vi "Init.vi"(8 "error in":errorcluster, 10 "Sourcegrid Container":refnum<k24>(container), 11 "PDO Grid in":refnum<class "PDO Grid.lvclass">) -> (0 "error out":errorcluster, 3 "PDO Grid out":refnum<class "PDO Grid.lvclass">)   [LabVIEW 2019, in "PDO Grid.lvlib" / "PDO Grid.lvclass"]
uses:
  PDO Grid.lvclass
  D:/git/Sourcegrid-LabVIEW/source/Grid/SourceGrid.lvclass
  D:/git/Sourcegrid-LabVIEW/dll/SourceGrid.dll
  Sourcegrid-LabVIEW/dll/SourceGrid.dll
  PDO Mapping ColumnHeader/PDO Mapping Column Header.lvclass
  D:/git/Sourcegrid-LabVIEW/source/Cells/Cell/Cell.lvclass
  Sourcegrid-LabVIEW/source/Grid/SourceGrid.lvclass
  Sourcegrid-LabVIEW/source/System.Drawing.Color.ctl
  Sourcegrid-LabVIEW/source/SourceGrid.lvlib
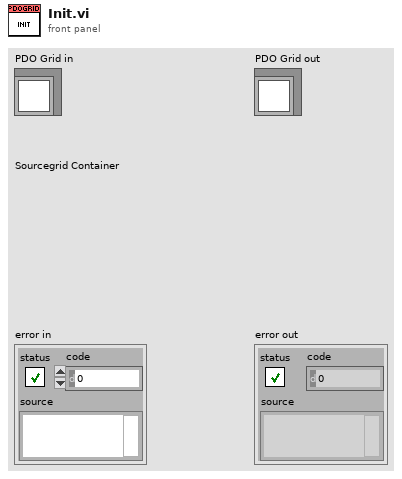
[diagram p1: front panel]
types:
  T1 = typedef "SourceGrid.lvlib/System.Drawing.Color.ctl" = enum16{"AliceBlue", "AntiqueWhite", "Aqua", "Aquamarine", "Azure", "Beige", "Bisque", "Black", "BlanchedAlmond", "Blue", "BlueViolet", "Brown", "BurlyWood", "CadetBlue", "Chartreuse", "Chocolate", "Coral", "CornflowerBlue", "Cornsilk", "Crimson", "Cyan", "DarkBlue", "DarkCyan", "DarkGoldenrod", "DarkGray", "DarkGreen", "DarkKhaki", "DarkMagenta", "DarkOliveGreen", "DarkOrange", "DarkOrchid", "DarkRed", "DarkSalmon", "DarkSeaGreen", "DarkSlateBlue", "DarkSlateGray", "DarkTurquoise", "DarkViolet", "DeepPink", "DeepSkyBlue", "DimGray", "DodgerBlue", "Firebrick", "FloralWhite", "ForestGreen", "Fuchsia", "Gainsboro", "GhostWhite", "Gold", "Goldenrod", "Gray", "Green", "GreenYellow", "Honeydew", "HotPink", "IndianRed", "Indigo", "Ivory", "Khaki", "Lavender", "LavenderBlush", "LawnGreen", "LemonChiffon", "LightBlue", "LightCoral", "LightCyan", "LightGoldenrodYellow", "LightGray", "LightGreen", "LightPink", "LightSalmon", "LightSeaGreen", "LightSkyBlue", "LightSlateGray", "LightSteelBlue", "LightYellow", "Lime", "LimeGreen", "Linen", "Magenta", "Maroon", "MediumAquamarine", "MediumBlue", "MediumOrchid", "MediumPurple", "MediumSeaGreen", "MediumSlateBlue", "MediumSpringGreen", "MediumTurquoise", "MediumVioletRed", "MidnightBlue", "MintCream", "MistyRose", "Moccasin", "NavajoWhite", "Navy", "OldLace", "Olive", "OliveDrab", "Orange", "OrangeRed", "Orchid", "PaleGoldenrod", "PaleGreen", "PaleTurquoise", "PaleVioletRed", "PapayaWhip", "PeachPuff", "Peru", "Pink", "Plum", "PowderBlue", "Purple", "Red", "RosyBrown", "RoyalBlue", "SaddleBrown", "Salmon", "SandyBrown", "SeaGreen", "SeaShell", "Sienna", "Silver", "SkyBlue", "SlateBlue", "SlateGray", "Snow", "SpringGreen", "SteelBlue", "Tan", "Teal", "Thistle", "Tomato", "Transparent", "Turquoise", "Violet", "Wheat", "White", "WhiteSmoke", "Yellow"}
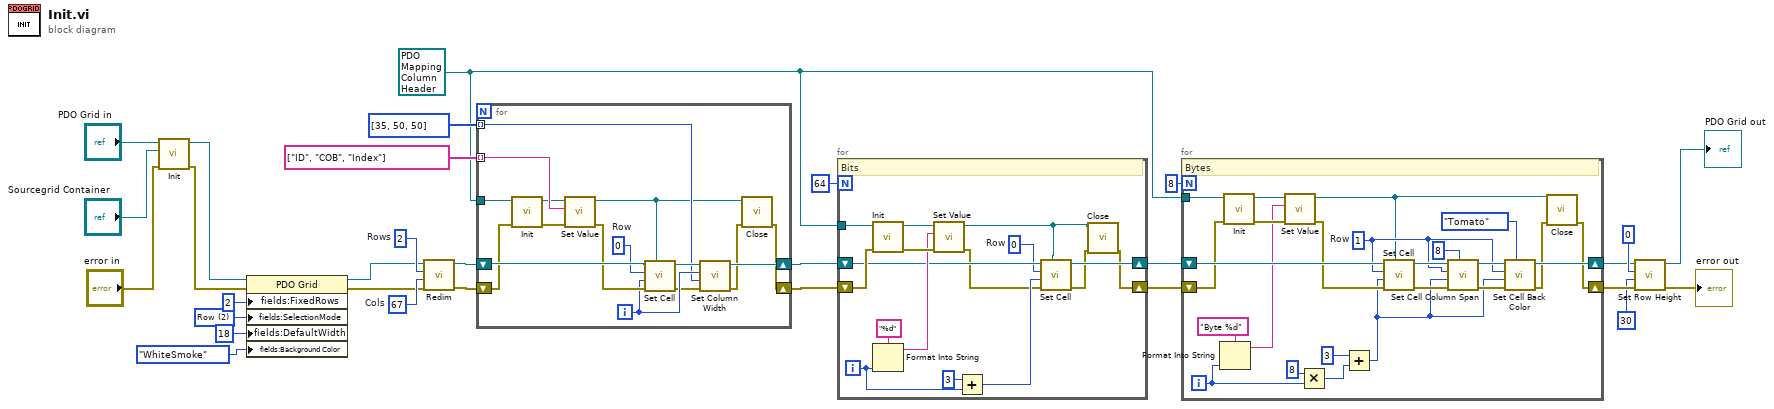
[diagram p0: block diagram]
diagram:
  w1 = refnum<class "PDO Mapping Column Header.lvclass"> refnum ("UI Actor.lvlib:PDOMapping ColumnHeader.lvclass")
  w28 = 2 items=["Cell"=1, "Row"=2, "Column"=3] ("SelectionMode")
  w29 = 67  # Cols
  w30 = 2  # Rows
  n1 = call-parent "Init.vi"("error in"="error in", "Sourcegrid Container"="Sourcegrid Container", "Grid in"="PDO Grid in") -> ("error out"=w4:errorcluster, "Grid out"=w7:refnum<class "PDO Grid.lvclass">)  [unwired: 7 in]
  n2 = property class="PDO Grid"(reference=w7, error in=w4, "fields:FixedRows"=2 ("FixedRows"), "fields:SelectionMode"=w28, "fields:DefaultWidth"=18 ("DefaultWidth"), "fields:Background Color"=System.Drawing.Color."WhiteSmoke" ("Color")) -> (reference out=w23:refnum<class "PDO Grid.lvclass">, error out=w21:errorcluster)
  n3 = call "Redim.vi"("error in"=w21, "Columns"=w29, "Rows"=w30, "Sourcegrid in"=w23) -> ("error out"=w20:errorcluster, "Sourcegrid out"=w22:refnum<class "PDO Grid.lvclass">)  [unwired: 6 in]
  n4 = for {
    shift-right: [w32] -> w18
    shift-left: w20 -> [w44]
    shift-right: [w41] -> w17
    shift-left: w22 -> [w46]
    tunnel: string[] ["ID", "COB", "Index"] -> [w38] mode=indexing
    tunnel: w1 -> [w36]
    tunnel: i32[] [35, 50, 50] -> [w39] mode=indexing
    i -> [w40]
    w45 = 0  # Row
    n5 = call-dynamic "Init.vi"("error in"=w44, "PDO Mapping Column Header in"=w36) -> ("error out"=w37:errorcluster, "PDO Mapping Column Header out"=w35:refnum<class "PDO Mapping Column Header.lvclass">)  [unwired: 8 in]
    n6 = call-dynamic "Set Value.vi"("error in"=w37, "Value"=w38, "PDO Mapping Column Header in"=w35) -> ("error out"=w43:errorcluster, "PDO Mapping Column Header out"=w31:refnum<class "PDO Mapping Column Header.lvclass">)  [unwired: 7 in]
    n7 = call "Set Cell.vi"("Cell"=w31, "error in"=w43, "Column"=w40, "Row"=w45, "Sourcegrid in"=w46) -> ("error out"=w34:errorcluster, "Sourcegrid out"=w42:refnum<class "PDO Grid.lvclass">)  [unwired: 5 in]
    n8 = call "Set Column Width.vi"("error in"=w34, "Width"=w39, "Column"=w40, "Sourcegrid in"=w42) -> ("error out"=w33:errorcluster, "Sourcegrid out"=w41:refnum<class "PDO Grid.lvclass">)  [unwired: 6 in]
    n9 = call-dynamic "Close.vi"("error in"=w33, "Cell in"=w31) -> ("error out"=w32:errorcluster)  [unwired: 8 in, 1 out]
  }
  n10 = for {
    N: 64 -> [_]
    shift-right: [w48] -> w10
    shift-left: w18 -> [w61]
    shift-right: [w55] -> w9
    shift-left: w17 -> [w54]
    tunnel: w1 -> [w50]
    i -> [w56]
    w53 = 0  # Row
    # "Bits"
    n11 = call-dynamic "Init.vi"("error in"=w61, "PDO Mapping Column Header in"=w50) -> ("error out"=w60:errorcluster, "PDO Mapping Column Header out"=w59:refnum<class "PDO Mapping Column Header.lvclass">)  [unwired: 8 in]
    n12 = Format Into String(format string="%d", w56) -> (resulting string=w58:string)  [unwired: 2 in, 1 out]
    n13 = call-dynamic "Set Value.vi"("error in"=w60, "Value"=w58, "PDO Mapping Column Header in"=w59) -> ("error out"=w51:errorcluster, "PDO Mapping Column Header out"=w47:refnum<class "PDO Mapping Column Header.lvclass">)  [unwired: 7 in]
    n14 = Add(x=3, y=w56) -> (x+y=w52:i32)
    n15 = call "Set Cell.vi"("Cell"=w47, "error in"=w51, "Column"=w52, "Row"=w53, "Sourcegrid in"=w54) -> ("error out"=w49:errorcluster, "Sourcegrid out"=w55:refnum<class "PDO Grid.lvclass">)  [unwired: 5 in]
    n16 = call-dynamic "Close.vi"("error in"=w49, "Cell in"=w47) -> ("error out"=w48:errorcluster)  [unwired: 8 in, 1 out]
  }
  n17 = for {
    N: 8 -> [_]
    shift-right: [w64] -> w16
    shift-left: w10 -> [w82]
    shift-right: [w71] -> w3
    shift-left: w9 -> [w85]
    tunnel: w1 -> [w66]
    i -> [w78]
    w68 = 1  # Row
    # "Bytes"
    n18 = Format Into String(format string="Byte %d", w78) -> (resulting string=w76:string)  [unwired: 2 in, 1 out]
    n19 = call-dynamic "Init.vi"("error in"=w82, "PDO Mapping Column Header in"=w66) -> ("error out"=w81:errorcluster, "PDO Mapping Column Header out"=w84:refnum<class "PDO Mapping Column Header.lvclass">)  [unwired: 8 in]
    n20 = call-dynamic "Set Value.vi"("error in"=w81, "Value"=w76, "PDO Mapping Column Header in"=w84) -> ("error out"=w80:errorcluster, "PDO Mapping Column Header out"=w63:refnum<class "PDO Mapping Column Header.lvclass">)  [unwired: 7 in]
    n21 = Multiply(x=8, y=w78) -> (x*y=w75:i32)
    n22 = Add(x=3, y=w75) -> (x+y=w67:i32)
    n23 = call "Set Cell.vi"("Cell"=w63, "error in"=w80, "Column"=w67, "Row"=w68, "Sourcegrid in"=w85) -> ("error out"=w86:errorcluster, "Sourcegrid out"=w74:refnum<class "PDO Grid.lvclass">)  [unwired: 5 in]
    n24 = call "Set Cell Column Span.vi"("Range"=8, "error in"=w86, "Column"=w67, "Row"=w68, "SourceGrid in"=w74) -> ("error out"=w70:errorcluster, "SourceGrid out"=w72:refnum<class "PDO Grid.lvclass">)  [unwired: 5 in]
    n25 = call "Set Cell Back Color.vi"("Color"=System.Drawing.Color."Tomato", "error in"=w70, "Column"=w67, "Row"=w68, "SourceGrid in"=w72) -> ("error out"=w65:errorcluster, "SourceGrid out"=w71:refnum<class "PDO Grid.lvclass">)  [unwired: 5 in]
    n26 = call-dynamic "Close.vi"("error in"=w65, "Cell in"=w63) -> ("error out"=w64:errorcluster)  [unwired: 8 in, 1 out]
  }
  n27 = call "Set Row Height.vi"("error in"=w16, "Height"=30, "Row"=0, "SourceGrid in"=w3) -> ("error out"=→"error out":errorcluster, "SourceGrid out"=→"PDO Grid out":refnum<class "PDO Grid.lvclass">)  [unwired: 6 in]
